vi "Trim_Meas_ODFT_iHV.vi"(10 "Ext_HV":dbl=38.0 format="%#_13g", 11 "Semiconductor Module Context":T1) -> (0 "error out":errorcluster, 3 "ODFT_Meas":dbl format="%#_6p")   [LabVIEW 2013]
uses:
  <vilib>/NI_TestStand_SemiconductorModule/NI_TestStand_Semiconductor_Module.lvlibp/PinMap/General/SemiconductorModuleContext.ctl
  <instrlib>/niHSDIO/niHSDIO.llb/niHSDIO_ctl Trigger Script - trigID Values (Ring).ctl
  <vilib>/NI_TestStand_SemiconductorModule/NI_TestStand_Semiconductor_Module.lvlibp/PinMap/DC Power/PinsToNIDCPowerSessions.vi
  <vilib>/NI_TestStand_SemiconductorModule/NI_TestStand_Semiconductor_Module.lvlibp
panel:
  in  "Pins":string[](array[string])=["HV"]
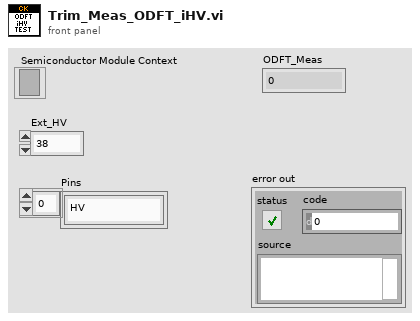
[diagram p1: front panel]
types:
  T1 = typedef "NI_TestStand_Semiconductor_Module.lvlibp/SemiconductorModuleContext.ctl" = refnum<k7>
  T2 = typedef "niHSDIO_ctl Trigger Script - trigID Values (Ring).ctl" = string
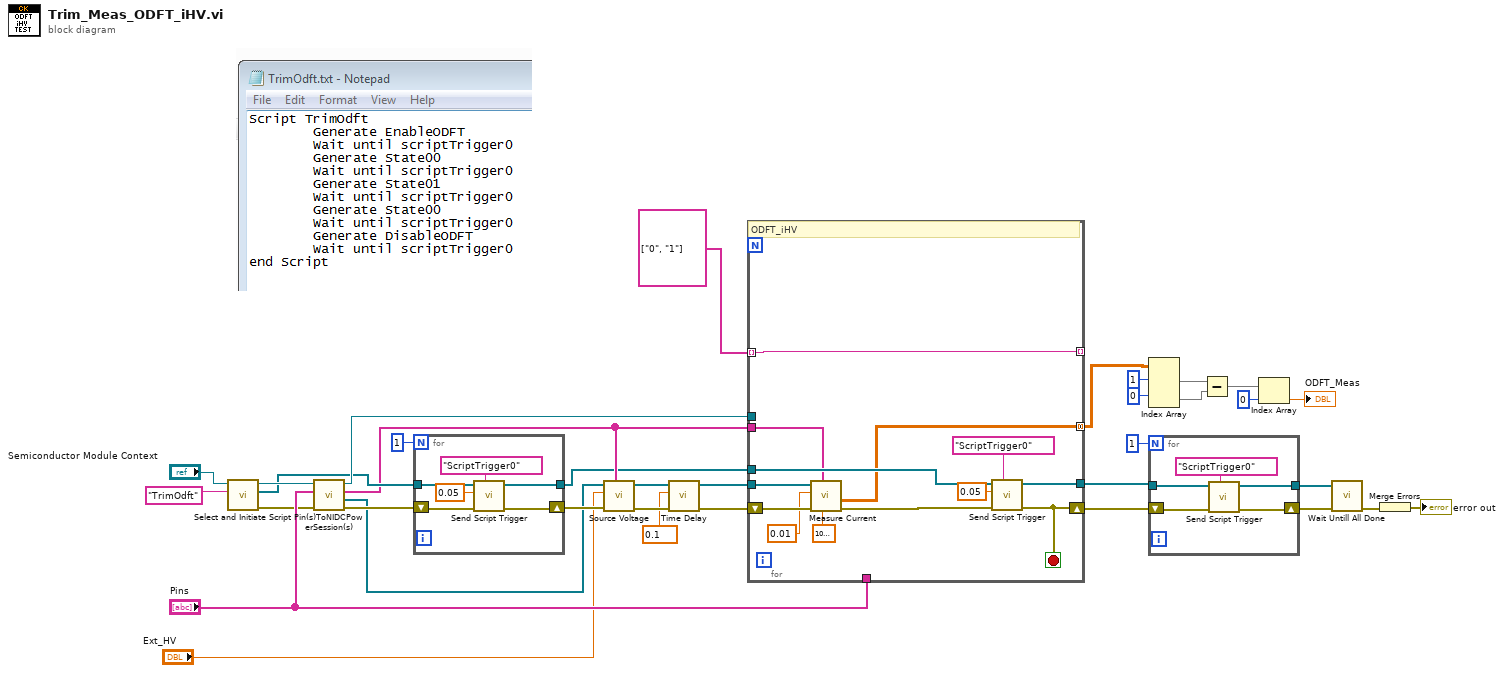
[diagram p0: block diagram]
diagram:
  n1 = call "Select and Initiate Script.vi"("script name"="TrimOdft", "Semiconductor Module Context"="Semiconductor Module Context") -> ("error out"=w22:errorcluster, "HSDIO GEN Sessions Out"=w23:refnum<k15>[], "Semiconductor Module Context Out"=w24:T1)  [unwired: 7 in]
  n2 = call-poly <vilib>:"Pin(s)ToNIDCPowerSession(s).vi"("error in (no error)"=w22, "Pins"="Pins", "Semiconductor Module Context"=w24) -> ("error out"=w33:errorcluster, "Instrument Sessions"=w21:refnum<k15>[], "Channel Lists"=w20:string[], "Semiconductor Module Context Out"=w26:T1)  [unwired: 4 in, 1 out]
  n3 = for {
    N: 1 -> [_]
    shift-right: [w38] -> w31
    shift-left: w33 -> [w39]
    tunnel: w23 -> [w37]
    tunnel: [w36] -> w18
    n4 = call "Send Script Trigger.vi"("trigger id (script trigger 0)"=T2 "ScriptTrigger0", "error in (no error)"=w39, "Delay Time (s)"=0.05, "HSDIO Sessions In"=w37) -> ("error out"=w38:errorcluster, "HSDIO Sessions Out"=w36:refnum<k15>[])  [unwired: 6 in]
  }
  n5 = call "Source Voltage.vi"("Channel Lists"=w20, "error in (no error)"=w31, "voltage level"="Ext_HV", "Instrument Sessions In"=w21) -> ("error out"=w17:errorcluster, "Instrument Sessions Out"=w30:refnum<k15>[])  [unwired: 4 in, 2 out]
  n6 = call "Time Delay"("error in (no error)"=w17, "Delay Time (s)"=0.1) -> ("error out"=w16:errorcluster)  [unwired: 9 in]
  n7 = for {
    tunnel: string[] ["0", "1"] -> [w53] mode=indexing
    tunnel: w30 -> [w47]
    tunnel: w26 -> [_]
    shift-right: [w50] -> w4
    shift-left: w16 -> [w48]
    tunnel: [w53] -> _ mode=indexing
    tunnel: "Pins" -> [_]
    tunnel: w18 -> [w51]
    tunnel: w20 -> [w46]
    tunnel: [w49] -> w11 mode=concatenating
    tunnel: [w43] -> w3
    stop <- w50 stop-if-true
    # "ODFT_iHV"
    n8 = call "Measure Current.vi"("Result Multiplier"=1000000.0, "Channel Lists"=w46, "error in (no error)"=w48, "Delay Time (s)"=0.01, "DCPower Sessions In"=w47) -> ("error out"=w41:errorcluster, "current measurements"=w49:dbl[][])  [unwired: 4 in, 1 out]
    n9 = call "Send Script Trigger.vi"("trigger id (script trigger 0)"=T2 "ScriptTrigger0", "error in (no error)"=w41, "Delay Time (s)"=0.05, "HSDIO Sessions In"=w51) -> ("error out"=w50:errorcluster, "HSDIO Sessions Out"=w43:refnum<k15>[])  [unwired: 6 in]
  }
  n10 = Index Array(array=w11, index (row) #1=1 ("index (row)"), index (row) #2=0 ("index (row)")) -> (element #1=w10:dbl[], element #2=w9:dbl[])  [unwired: 2 in]
  n11 = for {
    N: 1 -> [_]
    shift-right: [w56] -> w2
    shift-left: w4 -> [w57]
    tunnel: w3 -> [w55]
    tunnel: [w54] -> w1
    n12 = call "Send Script Trigger.vi"("trigger id (script trigger 0)"=T2 "ScriptTrigger0", "error in (no error)"=w57, "HSDIO Sessions In"=w55) -> ("error out"=w56:errorcluster, "HSDIO Sessions Out"=w54:refnum<k15>[])  [unwired: 7 in]
  }
  n13 = Subtract(x=w10, y=w9) -> (x-y=w8:dbl[])
  n14 = Index Array(array=w8, index=0) -> (element=→"ODFT_Meas":dbl)
  n15 = call "Wait Untill All Done.vi"("error in (no error)"=w2, "HSDIO Sessions In"=w1) -> ("error out"=w19:errorcluster)  [unwired: 8 in, 1 out]
  n16 = Merge Errors(w19) -> (→"error out":errorcluster)
